vi "Simple Execute.vi"() -> ()   [LabVIEW 2020]
uses:
  Engine/Engine.lvclass
  SequenceFile/SequenceFile.lvclass
  Report/Report.lvclass
panel:
  in  "Show Report?":bool
  in  "Entry Point":string(combo)="Single Pass"
  out "Status":string
  in  "SequenceFile Path":path=path "C:/Users/Public/Documents/National Instruments/TestStand 2019 (32-bit)/Examples/Demos/Computer Motherboard Test/LabVIEW/Computer Motherboard Test Sequence.seq"
  # "1."
  # "2."
  # "3."
  # "1. Select the sequence file you'd like to run.\n\n2. Enter the name of the entry point to use in the process model. This is usually 'Test UUTs' or 'Single Pass' for models that ship with TestStand.\n\n3. Choose whether to automatically display the report in an available viewer (Internet Explorer for ATML) when done."
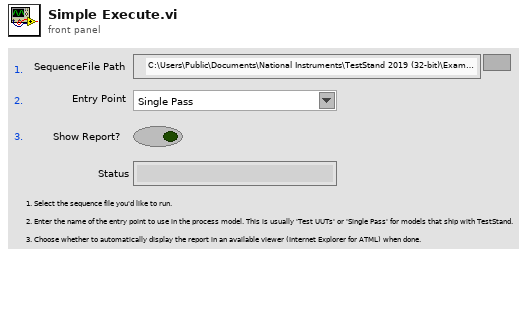
[diagram p1: front panel]
types:
  T1 = typedef "TSS.lvlib/Engine.lvclass/Session Handle.ctl" = refnum<data-value>
  T2 = typedef "TSS.lvlib/SequenceFile.lvclass/Session Handle.ctl" = refnum<data-value>
  T3 = typedef "TSS.lvlib/Report.lvclass/Session Handle.ctl" = refnum<data-value>
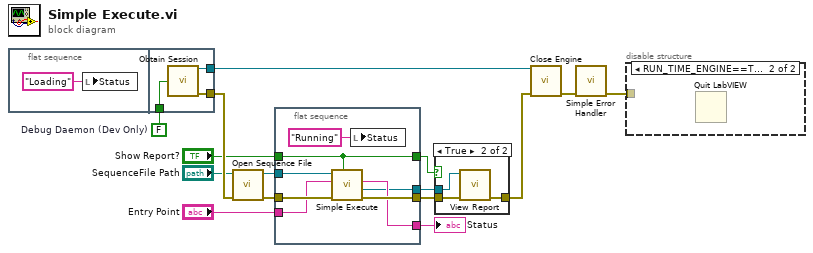
[diagram p0: block diagram]
diagram:
  w7 = FALSE  # Debug Daemon (Dev Only)
  n1 = flat-sequence {
    tunnel: [w19] -> w9
    tunnel: [w18] -> w15
    tunnel: w7 -> [w17]
    frame #0 {
      n2 = local write "Status"("Loading" ("Status")) -> ()
    }
    frame #1 {
      n3 = call "Obtain Session.vi"("Debug Daemon (Dev Only)"=w17) -> ("Session Handle"=w19:T1, "error out"=w18:errorcluster)  [unwired: 12 in, 1 out]
    }
  }
  n4 = call "Open Sequence File.vi"("error in (no error)"=w15, "Path"="SequenceFile Path") -> ("error out"=w10:errorcluster, "Session Handle out"=w8:T2)  [unwired: 8 in]
  n5 = flat-sequence {
    tunnel: w8 -> [w27]
    tunnel: w10 -> [w26]
    tunnel: "Entry Point" -> [w25]
    tunnel: [w24] -> w2
    tunnel: [w23] -> w12
    tunnel: "Show Report?" -> [w21]
    tunnel: [w21] -> w3
    tunnel: [w20] -> w4
    frame #0 {
      n6 = call "Simple Execute.vi"("Return Report? (F)"=w21, "error in (no error)"=w26, "Entry Point / Sequence"=w25, "Session Handle in"=w27) -> ("error out"=w24:errorcluster, "Report"=w20:T3, "Status"=w23:string)  [unwired: 4 in, 1 out]
      n7 = local write "Status"("Running" ("Status")) -> ()
    }
  }
  n8 = case shown="True" w3 {
    tunnel: w4 -> [_ w31]
    tunnel: w2 -> [w28 w30]
    tunnel: [w28 w29] -> w1
    frame False {
    }
    frame True {
      n9 = call "View Report.vi"("error in (no error)"=w30, "Report In"=w31) -> ("error out"=w29:errorcluster)  [unwired: 8 in, 1 out]
    }
  }
  n10 = call "Close Engine.vi"("Session Handle in"=w9, "error in (no error)"=w1) -> ("error out"=w14:errorcluster)  [unwired: 13 in]
  n11 = call <vilib>:"Simple Error Handler.vi"("error in (no error)"=w14) -> ("error out"=w6:errorcluster)  [unwired: 4 in, 4 out]
  n12 = disable-structure shown="RUN_TIME_ENGINE==True" {
    disable-tunnel: w6 -> [_ _]
    frame condition #0 (active) {
    }
    frame condition #1 {
      n13 = Quit LabVIEW() -> ()  [unwired: 1 in]
    }
  }
  "Status" <- w12
